vi "Read.vi"(8 "error in (no error)":errorcluster, 11 "Add To Var Command Config in":refnum<class "Add To Var Command Config.lvclass">) -> (0 "error out":errorcluster, 1 "Value":dbl, 2 "Variable":string, 3 "Add To Var Command Config out":refnum<class "Add To Var Command Config.lvclass">)   [LabVIEW 2020, in "VolatusSeqConfig.lvlib" / "Add To Var Command Config.lvclass"]
uses:
  Add To Var Command Config.lvclass
  Add To Var Command Config.lvclass/Add To Var Command Config.ctl
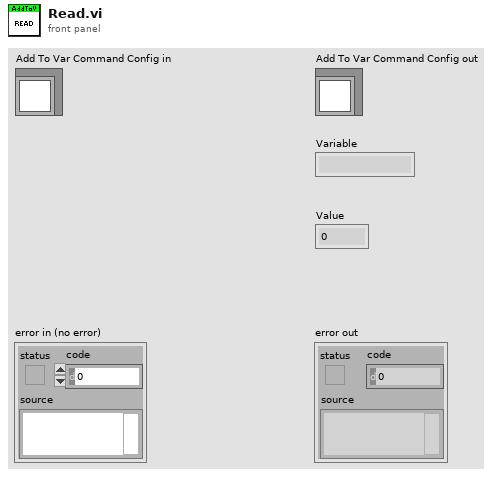
[diagram p1: front panel]
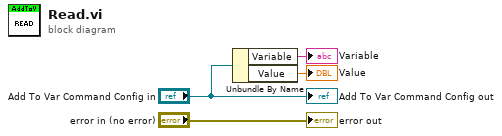
[diagram p0: block diagram]
diagram:
  n1 = Unbundle By Name("Add To Var Command Config in") -> ("Variable"=→"Variable":string, "Value"=→"Value":dbl)
  "error out" <- "error in (no error)"
  "Add To Var Command Config out" <- "Add To Var Command Config in"
